vi "Initialize PVs.vi"(7 "PV-Name-Suffix":string[](array[string]), 8 "error in (no error)":errorcluster, 9 "MultiplePVs":T1(array[cluster]), 10 "SinglePVs":cluster{"PV-Name":string, "PV-Type":string}[](array[cluster]), 11 "CS++BaseActor in":refnum<class "CS++BaseActor.lvclass">) -> (0 "error out":errorcluster, 1 "PVConnections-n":refnum<class "PVConnection.lvclass">[][](array[class]), 2 "PVConnections":refnum<class "PVConnection.lvclass">[](array[class]), 3 "CS++BaseActor out":refnum<class "CS++BaseActor.lvclass">, 5 "Found?":bool)   [LabVIEW 2015, in "CS++BaseActor.lvlib" / "CS++BaseActor.lvclass"]
doc: "This is a small help VI which should simplify the creation of an \"Initialize Attributes.vi\" for devices. As inputsit requires the URL lists of the PVs (1D and variables with channels) and returns the prepared connections."
uses:
  CS++BaseActor.lvclass
  Classes/CS++ProcessVariables/PVConnection/PVConnection.lvclass
  Classes/CS++ProcessVariables/ProcessVariable/PV.lvclass
  CS++BaseActor.lvclass/CS++BaseActor.ctl
  Classes/CS++ProcessVariables/ProcessVariable/PV.lvclass/PV.ctl
  Classes/CS++BaseClasses/Base/CS++Base.lvclass/CS++Base.ctl
  Classes/CS++ProcessVariables/ProcessVariable/Write Name.vi
  Classes/CS++ProcessVariables/ProcessVariable/Write PV URL.vi
  Classes/CS++ProcessVariables/ProcessVariable/Write Type Descriptor.vi
  <vilib>/Utility/error.llb/Error Cluster From Error Code.vi
  Classes/CS++BaseClasses/Factory/CS++Factory.lvclass
  Libraries/Utilities/CS++Utilities.lvlib
  Classes/CS++ProcessVariables/CS++ProcessVariables.lvlib
  Classes/CS++BaseClasses/Base/CS++Base.lvclass
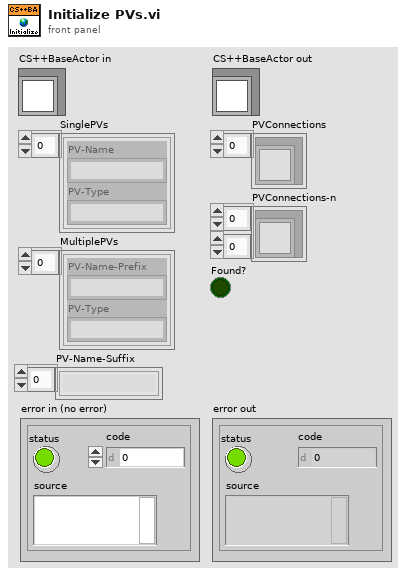
[diagram p1: front panel]
types:
  T1 = cluster{"PV-Name-Prefix":string, "PV-Type":string}[]
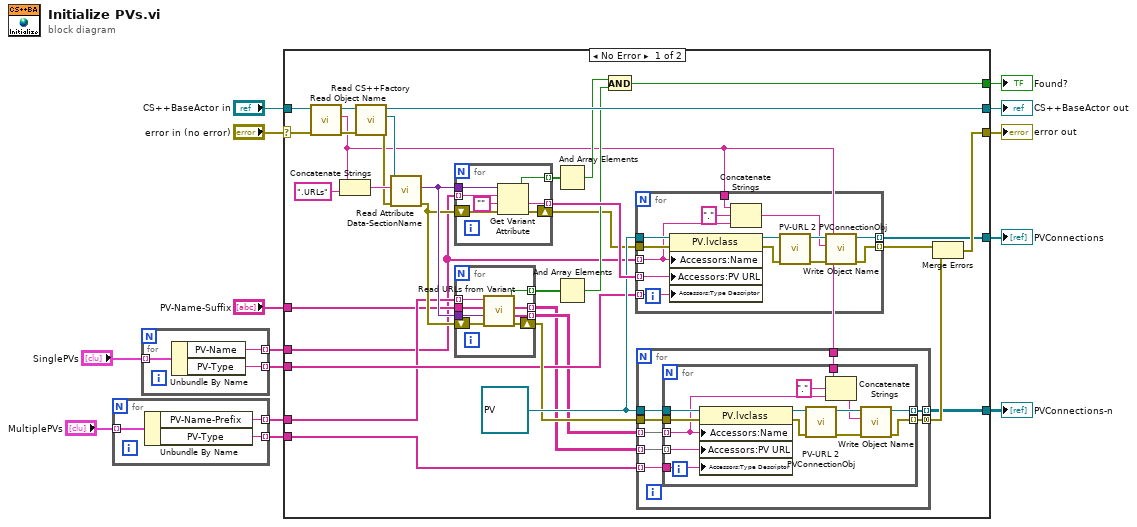
[diagram p0: block diagram]
diagram:
  n1 = for {
    tunnel: "MultiplePVs" -> [w17] mode=indexing
    tunnel: [w16] -> w2 mode=indexing
    tunnel: [w15] -> w1 mode=indexing
    n2 = Unbundle By Name(w17) -> ("PV-Name-Prefix"=w16:string, "PV-Type"=w15:string)
  }
  n3 = for {
    tunnel: "SinglePVs" -> [w20] mode=indexing
    tunnel: [w19] -> w5 mode=indexing
    tunnel: [w18] -> w4 mode=indexing
    n4 = Unbundle By Name(w20) -> ("PV-Name"=w19:string, "PV-Type"=w18:string)
  }
  n5 = case shown="No Error" "error in (no error)" {
    selector: "error in (no error)" -> [w34 w106]
    tunnel: [w33 w106] -> w13
    tunnel: [w47 w105] -> w11
    tunnel: "CS++BaseActor in" -> [w48 w105]
    tunnel: [w31 _] -> w10
    tunnel: [w30 _] -> w9
    tunnel: [w29 _] -> w8
    tunnel: w5 -> [w24 _]
    tunnel: w4 -> [w28 _]
    tunnel: w2 -> [w27 _]
    tunnel: "PV-Name-Suffix" -> [w26 _]
    tunnel: w1 -> [w25 _]
    frame No Error {
      w39 = refnum<class "PV.lvclass"> refnum ("CS++ProcessVariables.lvlib:PV.lvclass")
      n6 = call "Read Object Name.vi"("error in (no error)"=w34, "CS++BaseActor in"=w48) -> ("error out"=w50:errorcluster, "Object Name"=w21:string, "CS++BaseActor out"=w49:refnum<class "CS++BaseActor.lvclass">)  [unwired: 7 in]
      n7 = Concatenate Strings(w21, ".URLs" ("string")) -> (w52:string)
      n8 = call "Read CS++Factory.vi"("error in (no error)"=w50, "CS++BaseActor in"=w49) -> ("error out"=w32:errorcluster, "CS++Factory"=w53:refnum<class "CS++Factory.lvclass">, "CS++BaseActor out"=w47:refnum<class "CS++BaseActor.lvclass">)  [unwired: 7 in]
      n9 = call-dynamic "Read Attribute Data-SectionName.vi"("error in (no error)"=w32, "Object Name"=w52, "CS++Factory in"=w53) -> ("error out"=w43:errorcluster, "Attribute Data"=w44:variant)  [unwired: 6 in, 1 out]
      n10 = for {
        tunnel: w24 -> [w101] mode=indexing
        tunnel: w44 -> [w102]
        shift-right: [w104] -> w38
        shift-left: w43 -> [w103]
        tunnel: [w100] -> w46 mode=indexing
        tunnel: [w98] -> w42 mode=indexing
        n11 = Get Variant Attribute(Variant=w102, name=w101, default value (empty Variant)="", error in=w103) -> (found=w100:bool, value=w98:string, error out=w104:errorcluster)  [unwired: 1 out]
      }
      n12 = for {
        tunnel: w27 -> [w97] mode=indexing
        tunnel: [w96] -> w45 mode=indexing
        tunnel: w44 -> [w94]
        tunnel: w26 -> [w93]
        tunnel: [w92] -> w22 mode=indexing
        shift-right: [w95] -> w37
        shift-left: w43 -> [w91]
        tunnel: [w90] -> w23 mode=indexing
        n13 = call "Read URLs from Variant.vi"("Error In"=w91, "URL Section Data"=w94, "Channel Names"=w93, "URL Prefix"=w97) -> ("Error Out"=w95:errorcluster, "Channel Names out"=w90:string[], "URLs"=w92:string[], "Found?"=w96:bool)  [unwired: 4 in]
      }
      n14 = And Array Elements(Boolean array=w46) -> (logical AND=w41:bool)
      n15 = And Array Elements(Boolean array=w45) -> (logical AND=w40:bool)
      n16 = And(x=w41, y=w40) -> (x .and. y?=w29:bool)
      n17 = for {
        tunnel: w39 -> [w88]
        tunnel: w42 -> [w80] mode=indexing
        tunnel: [w83] -> w31 mode=indexing
        tunnel: w28 -> [w85] mode=indexing
        tunnel: w38 -> [w86]
        tunnel: [w81] -> w36 mode=indexing
        tunnel: w24 -> [w77] mode=indexing
        tunnel: w21 -> [w78]
        n18 = property class="PV.lvclass"(reference=w88, error in=w86, "Accessors:Name"=w77, "Accessors:PV URL"=w80, "Accessors:Type Descriptor"=w85) -> (reference out=w89:refnum<class "PV.lvclass">, error out=w87:errorcluster)
        n19 = Concatenate Strings(w78, "." ("string"), w77) -> (w76:string)
        n20 = call "PV-URL 2 PVConnectionObj.vi"("Error In"=w87, "PV"=w89) -> ("Error Out"=w82:errorcluster, "PVConnection"=w84:refnum<class "PVConnection.lvclass">)  [unwired: 7 in, 1 out]
        n21 = call "Write Object Name.vi"("error in (no error)"=w82, "Object Name"=w76, "Base in"=w84) -> ("error out"=w81:errorcluster, "Base out"=w83:refnum<class "PVConnection.lvclass">)  [unwired: 7 in]
      }
      n22 = for {
        tunnel: w39 -> [w61]
        tunnel: w37 -> [w60]
        tunnel: w25 -> [w59] mode=indexing
        tunnel: w23 -> [w58] mode=indexing
        tunnel: [w57] -> w30 mode=indexing
        tunnel: [w56] -> w35 mode=concatenating
        tunnel: w22 -> [w55] mode=indexing
        tunnel: w21 -> [w54]
        n23 = for {
          tunnel: w61 -> [w74]
          tunnel: w58 -> [w63] mode=indexing
          tunnel: [w66] -> w57 mode=indexing
          tunnel: w59 -> [w71]
          tunnel: [w63] -> _ mode=indexing
          tunnel: w60 -> [w72]
          tunnel: [w68] -> w56 mode=indexing
          tunnel: w55 -> [w70] mode=indexing
          tunnel: w54 -> [w62]
          n24 = property class="PV.lvclass"(reference=w74, error in=w72, "Accessors:Name"=w63, "Accessors:PV URL"=w70, "Accessors:Type Descriptor"=w71) -> (reference out=w75:refnum<class "PV.lvclass">, error out=w73:errorcluster)
          n25 = call "PV-URL 2 PVConnectionObj.vi"("Error In"=w73, "PV"=w75) -> ("Error Out"=w69:errorcluster, "PVConnection"=w67:refnum<class "PVConnection.lvclass">)  [unwired: 7 in, 1 out]
          n26 = Concatenate Strings(w62, "." ("string"), w63) -> (w64:string)
          n27 = call "Write Object Name.vi"("error in (no error)"=w69, "Object Name"=w64, "Base in"=w67) -> ("error out"=w68:errorcluster, "Base out"=w66:refnum<class "PVConnection.lvclass">)  [unwired: 7 in]
        }
      }
      n28 = Merge Errors(w36, w35) -> (w33:errorcluster)
    }
    frame Error {
    }
  }
  "error out" <- w13
  "CS++BaseActor out" <- w11
  "PVConnections" <- w10
  "PVConnections-n" <- w9
  "Found?" <- w8
